vi "GUI.vi"() -> ()   [LabVIEW 2019]
uses:
  Histogram/Histogram.lvlib
panel:
  out "STATUS":u32
  out "BUSY":bool
  in  "CONNECT":bool
  in  "Tab Control":enum32{"ADC and Decimator", "pAmp CTRL"}(tab)
  in  "Full Scale Range":bool
  in  "DDR":bool
  in  "DCLK_RST":bool
  in  "ON":bool=TRUE
  in  "LED 1":bool
  in  "LED 0":bool=TRUE
  in  "CAL":bool
  in  "CAL_DLY":bool
  in  "OUTV":bool
  out "ADC500_CFG":u32=128
  in  "N":u32=100
  out "number":u32=9
  in  "SET POTS":bool
  in  "FINE OFFSET":u16(slide)=1023 scale=0.0..1023.0
  in  "OFFSET":u16(slide)=1023 scale=0.0..1023.0
  in  "HV_CTRL":bool
  out "RANGE 2":bool=TRUE
  out "RANGE 1":bool
  in  "RANGE":bool
  in  "LED":bool=TRUE
  in  "INIT":bool
  out "CONNECTED":bool
  in  "remote port or service name":u16=7
  in  "address":string="10.47.1.10"
  in  "Tab Control 2":T1(tab)
  in  "SET":bool
  in  "TRIGGER_LEVEL":u32=1200
  in  "TRIG_DELAY":u32=500
  in  "FIFO_SIZE":u32=1000
  in  "Trigger Edge":u32(ring)=2 items=["Falling Edge", "Rising Edge", "Auto", "EXT"]
  out "Oscilloscope":u32[](graph)
  in  "CONTINOUS":bool
  in  "Counts":u32
  in  "GEN HISTO":bool
  in  "ENABLE":bool
  out "HISTOGRAM":u32[](graph)
  out "DONE":bool
  out "Progress":u32(slide) max=100000 scale=-1.0..100000.0
  out "IMON GRAPH":dbl(graph)
  out "IMON":fxp<+,16,16>
  out "VMON":fxp<+,32,32>
  in  "VSET":u16
  in  "ON/OFF":bool
  in  "KILL":bool
  in  "TUPRMP":u16
  in  "TDRMP":u16
  out "VMON GRAPH":dbl(graph)
  out "VsetCoeff":dbl
  in  "VMAX":dbl
  out "pAs_STATUS":u8[](array[numeric])=[1, 0, 0, 0, 9, 0, 0, 0]
  out "PAM_INIT_STATUS":u8[](array[numeric])
  out "ADC500_STATUS":u8[](array[numeric])
  out "DEC_STATUS":u8[](array[numeric])
  out "nCoeff":dbl
  out "dacNVSET":u32
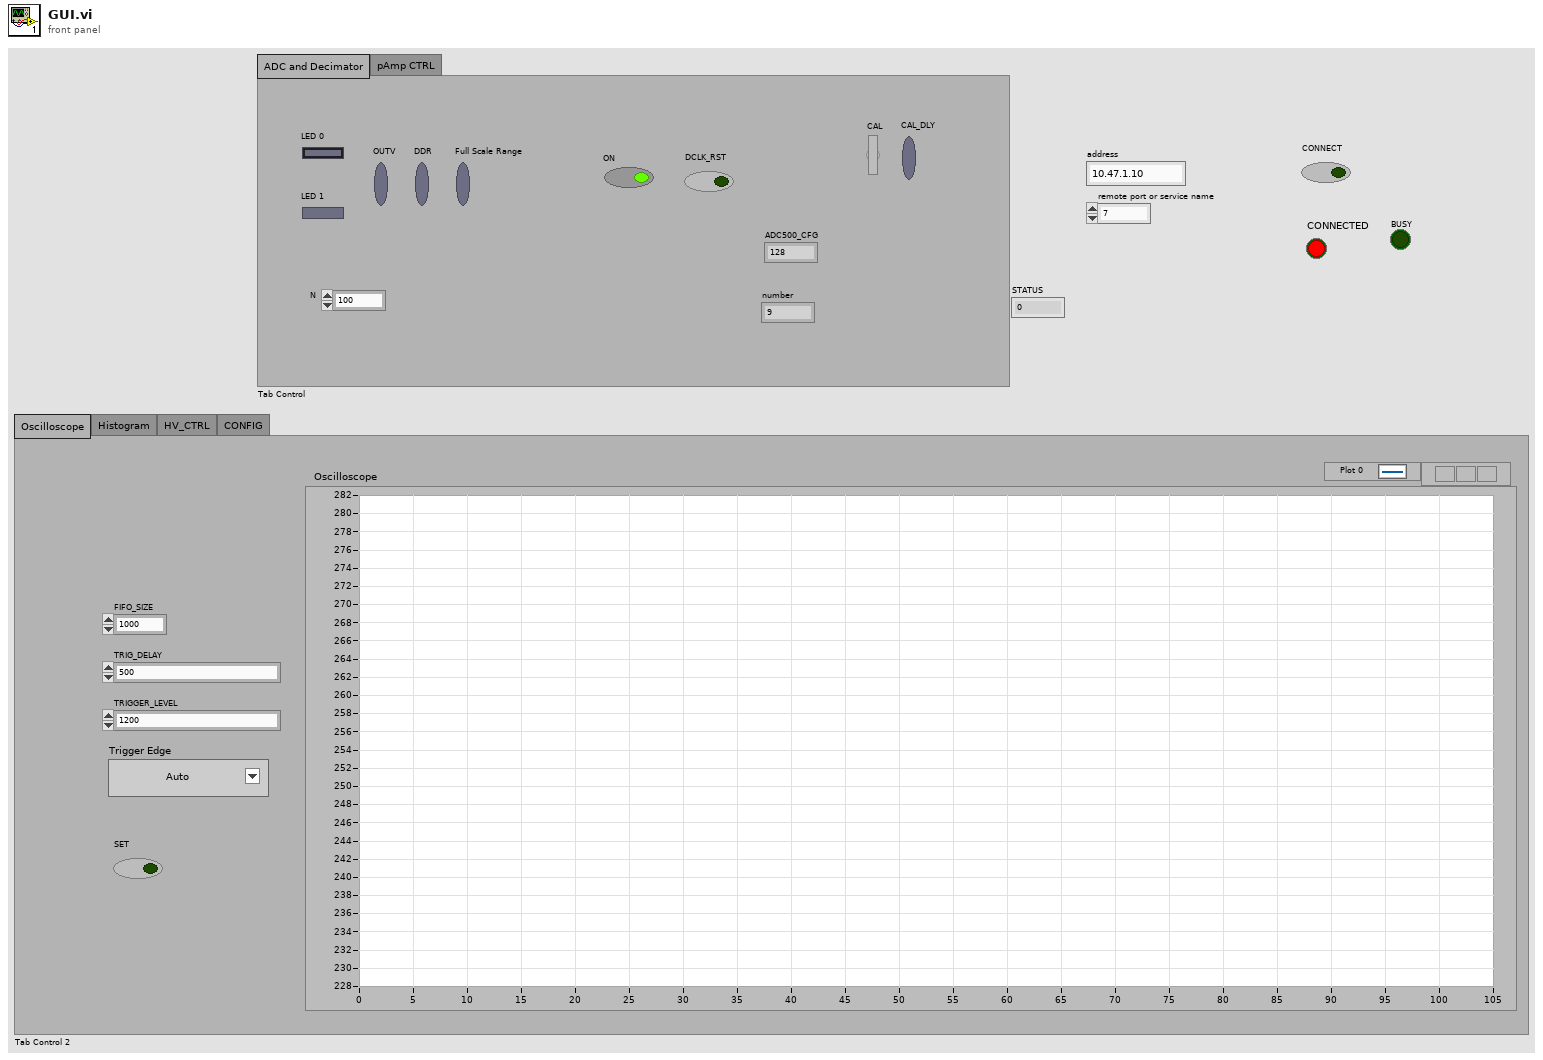
[diagram p1: front panel]
types:
  T1 = enum32{"Oscilloscope", "Histogram", "HV_CTRL", "CONFIG"}
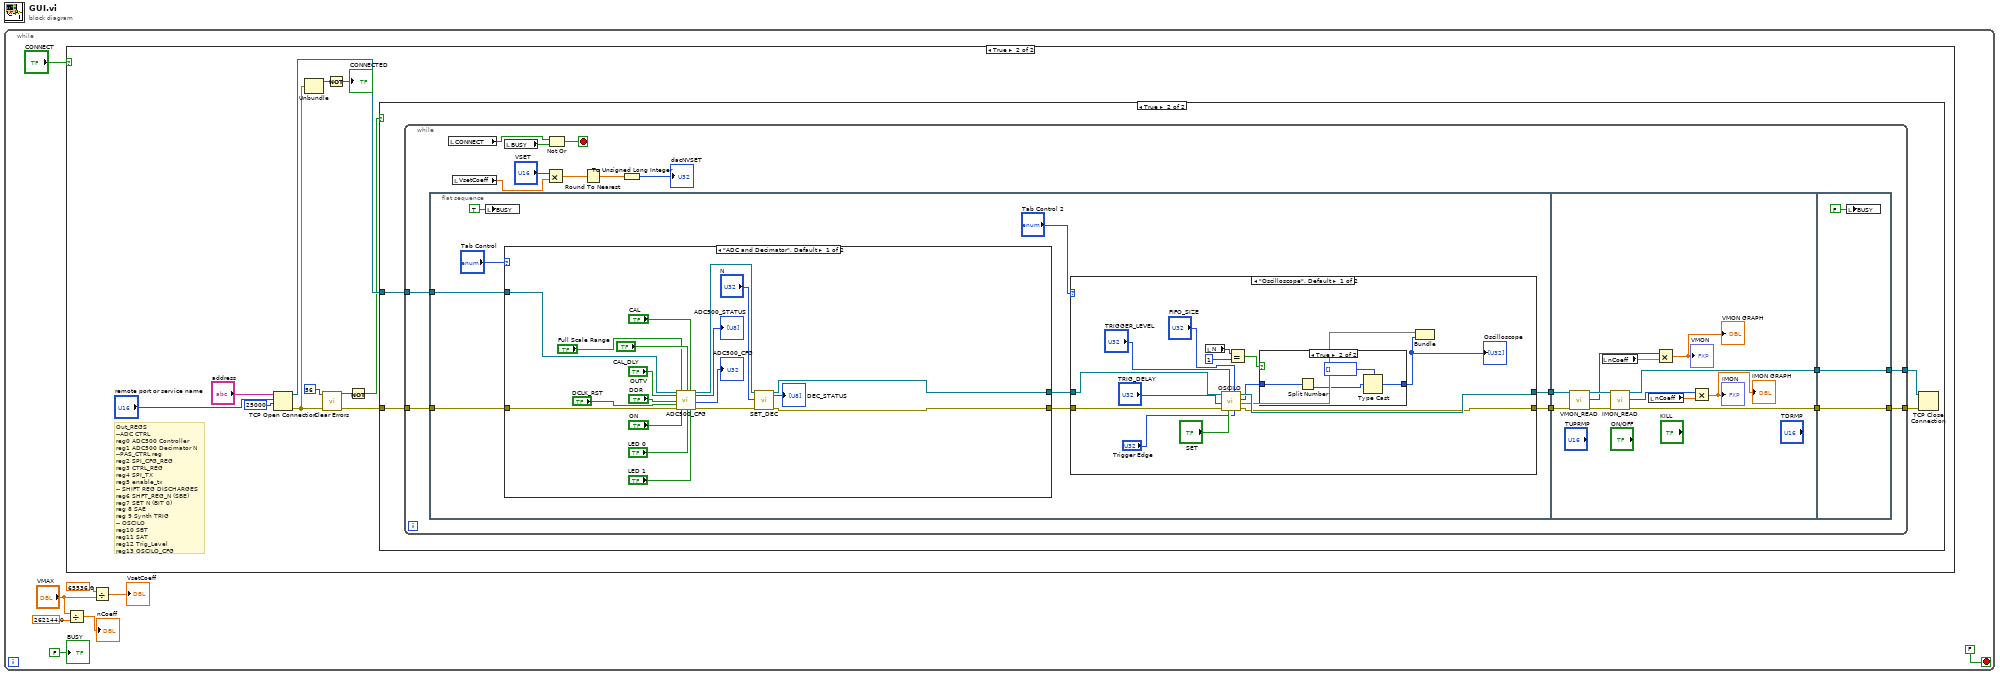
[diagram p0: block diagram]
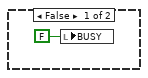
[diagram p3: hidden frame]
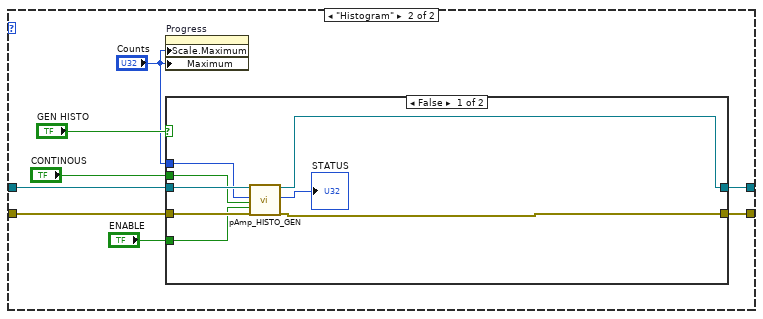
[diagram p5: hidden frame]
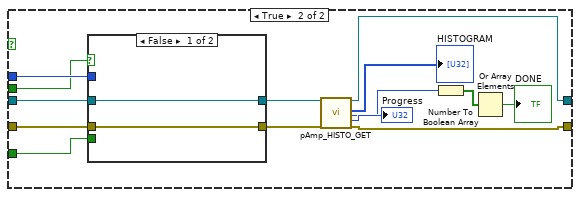
[diagram p6: hidden frame]
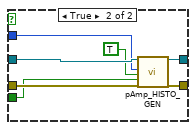
[diagram p7: hidden frame]
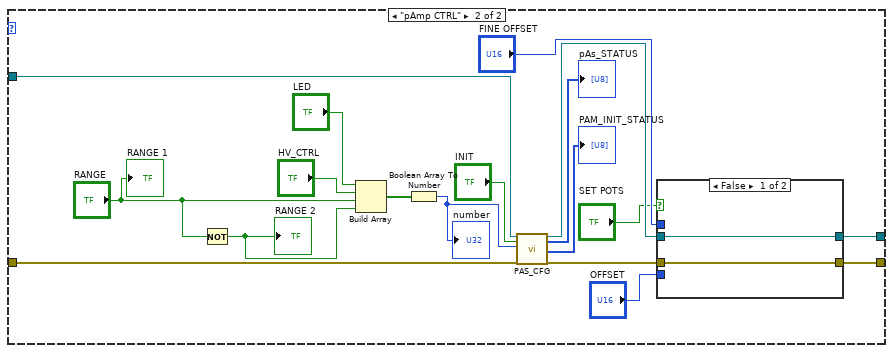
[diagram p8: hidden frame]
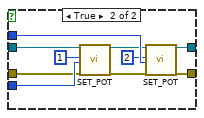
[diagram p9: hidden frame]
diagram:
  n1 = while {
    stop <- FALSE stop-if-true
    n2 = case shown="True" "CONNECT" {
      frame False {
      }
      frame True {
        # "Out_REGS\n--ADC CTRL\nreg0 ADC500 Controller\nreg1 ADC500 Decimator N\n--PAS_CTRL reg\nreg2 SPI_CFG_REG\nreg3 CTRL_REG\nreg4 SPI_TX\nreg5 enable_tx\n-- SHIFT REG DISCHARGES\nreg6 SHFT_REG_N (SBE)\nreg7 SET N (BIT 0)\nreg 8 SAE\nreg 9 Synth TRIG\n-- OSCILO \nreg10 SBT\nreg11 SAT\nreg12 Trig_Level\nreg13 OSCILO_CFG"
        n3 = TCP Open Connection(address="address", remote port or service name="remote port or service name", timeout ms (60000)=25000) -> (connection ID=w19:refnum<k5>, error out=w13:errorcluster)  [unwired: 2 in]
        n4 = Unbundle(w13) -> ("status"=w18:bool)  [unwired: 2 out]
        n5 = call <vilib>:"Clear Errors.vi"("error in (no error)"=w13, "specific error code to clear (0: all)"=56) -> ("error out"=w11:errorcluster, "specific error cleared?"=w10:bool)  [unwired: 4 in]
        n6 = Not(x=w18) -> (.not. x?=→"CONNECTED":bool)
        n7 = Not(x=w10) -> (.not. x?=w9:bool)
        n8 = case shown="True" w9 {
          tunnel: w19 -> [_ w24]
          tunnel: w11 -> [_ w23]
          frame False {
            n9 = local write "BUSY"(FALSE ("BUSY")) -> ()
          }
          frame True {
            n10 = while {
              tunnel: w24 -> [w40]
              tunnel: w23 -> [w39]
              tunnel: [w38] -> w21
              tunnel: [w37] -> w22
              stop <- w34 stop-if-true
              n11 = flat-sequence {
                tunnel: w40 -> [w49]
                tunnel: w39 -> [w48]
                tunnel: [w45] -> w33
                tunnel: [w44] -> w31
                tunnel: w33 -> [w167]
                tunnel: [w169] -> w32
                tunnel: w31 -> [w166]
                tunnel: [w168] -> w30
                tunnel: [w170] -> w37
                tunnel: [w172] -> w38
                tunnel: w32 -> [w172]
                tunnel: w30 -> [w170]
                frame #0 {
                  n12 = local write "BUSY"(TRUE) -> ()
                  n13 = case shown="\"ADC and Decimator\", Default" "Tab Control" {
                    tunnel: [w111 w131] -> w46
                    tunnel: [w109 w129] -> w42
                    tunnel: w48 -> [w127 w139]
                    tunnel: w49 -> [w126 w140]
                    frame "ADC and Decimator", Default {
                      n14 = call "ADC500_CFG.vi"("TCP Network Connection in"=w126, "OUTV"="OUTV", "DDR"="DDR", "DCLK_RST"="DCLK_RST", "error in (no error)"=w127, "Full Scale Range"="Full Scale Range", "ON"="ON", "CAL_DLY"="CAL_DLY", "LED 0"="LED 0", "CAL"="CAL", "LED 1"="LED 1") -> ("TCP Network Connection out"=w114:refnum<k5>, "ADC500_STATUS"=→"ADC500_STATUS":u8[], "ADC500_CFG"=→"ADC500_CFG":u32, "error out"=w112:errorcluster)  [unwired: 5 in]
                      n15 = call "SET_DEC.vi"("TCP Network Connection in"=w114, "N"="N", "error in (no error)"=w112) -> ("TCP Network Connection out"=w111:refnum<k5>, "DEC_STATUS"=→"DEC_STATUS":u8[], "error out"=w109:errorcluster)  [unwired: 14 in]
                    }
                    frame "pAmp CTRL" {
                      n16 = Not(x="RANGE") -> (.not. x?=w142:bool)
                      "RANGE 2" <- w142
                      n17 = Build Array("LED", "HV_CTRL", "RANGE", w142) -> (w141:bool[])
                      n18 = Boolean Array To Number(Boolean array=w141) -> (number=w138:u32)
                      "number" <- w138
                      n19 = call "PAS_CFG.vi"("TCP Network Connection in"=w140, "INIT"="INIT", "pAs_REG"=w138, "error in (no error)"=w139) -> ("TCP Network Connection out"=w132:refnum<k5>, "pAs_STATUS"=→"pAs_STATUS":u8[], "PAM_INIT"=→"PAM_INIT_STATUS":u8[], "error out"=w130:errorcluster)  [unwired: 12 in]
                      n20 = case shown="False" "SET POTS" {
                        tunnel: "OFFSET" -> [_ w157]
                        tunnel: "FINE OFFSET" -> [_ w156]
                        tunnel: w132 -> [w147 w153]
                        tunnel: [w147 w151] -> w131
                        tunnel: w130 -> [w146 w150]
                        tunnel: [w146 w148] -> w129
                        frame False {
                        }
                        frame True {
                          n21 = call "SET_POT.vi"("TCP Network Connection in"=w153, "POT_N"=u32 1, "VALUE"=w157, "error in (no error)"=w150) -> ("TCP Network Connection out"=w152:refnum<k5>, "error out"=w149:errorcluster)  [unwired: 13 in, 1 out]
                          n22 = call "SET_POT.vi"("TCP Network Connection in"=w152, "POT_N"=u32 2, "VALUE"=w156, "error in (no error)"=w149) -> ("TCP Network Connection out"=w151:refnum<k5>, "error out"=w148:errorcluster)  [unwired: 13 in, 1 out]
                        }
                      }
                      "RANGE 1" <- "RANGE"
                    }
                  }
                  n23 = case shown="\"Oscilloscope\", Default" "Tab Control 2" {
                    tunnel: w46 -> [w60 w77]
                    tunnel: [w59 w75] -> w45
                    tunnel: [w58 w74] -> w44
                    tunnel: w42 -> [w57 w76]
                    frame "Oscilloscope", Default {
                      n24 = local read "N"() -> (w54:u32)
                      n25 = call "OSCILO.vi"("Trigger Edge"="Trigger Edge", "FIFO_SIZE"="FIFO_SIZE", "SET"="SET", "TRIGGER_LEVEL"="TRIGGER_LEVEL", "error in (no error)"=w57, "TRIG_DELAY"="TRIG_DELAY", "TCP Network Connection in"=w60) -> ("error out"=w58:errorcluster, 1:w51, "Oscilloscope"=w55:u32[], "TCP Network Connection out"=w59:refnum<k5>)  [unwired: 1 in]
                      n26 = Equal?(x=w54, y=u32 1) -> (x = y?=w52:bool)
                      n27 = case shown="True" w52 {
                        tunnel: [w65 w68] -> w50
                        tunnel: w55 -> [w65 w67]
                        frame False {
                        }
                        frame True {
                          n28 = Split Number(x=w67) -> (lo(x)=w66:u16[])  [unwired: 1 out]
                          n29 = Type Cast(type=i8[] [] ("Oscilloscope"), x=w66) -> (*(type *) &x=w68:i8[])
                        }
                      }
                      "Oscilloscope" <- w50
                      n30 = Bundle(w51, "Oscilloscope"=w50) -> ()  [unwired: 1 in, 1 out]
                    }
                    frame "Histogram" {
                      n31 = property on="Progress" class="Slide (strict)"("Scale.Maximum"="Counts", "Maximum"="Counts") -> ()  [unwired: 2 in, 2 out]
                      n32 = case shown="False" "GEN HISTO" {
                        tunnel: w77 -> [w85 w89]
                        tunnel: w76 -> [w84 w90]
                        tunnel: [w79 w94] -> w75
                        tunnel: [w78 w93] -> w74
                        tunnel: "ENABLE" -> [w80 w86]
                        tunnel: "Counts" -> [w83 w88]
                        tunnel: "CONTINOUS" -> [w82 w87]
                        frame False {
                          n33 = call "pAmp_HISTO_GEN.vi"("TCP Network Connection in"=w85, "COUNTS"=w83, "CONTINOUS"=w82, "ENABLE"=w80, "error in (no error)"=w84) -> ("TCP Network Connection out"=w79:refnum<k5>, "STATUS"=→"STATUS":u32, "error out"=w78:errorcluster)  [unwired: 12 in]
                        }
                        frame True {
                          n34 = case shown="False" w87 {
                            tunnel: [w101 w108] -> w92
                            tunnel: [w100 w107] -> w91
                            tunnel: w90 -> [w100 w105]
                            tunnel: w89 -> [w101 w106]
                            tunnel: w88 -> [_ w104]
                            tunnel: w86 -> [_ w102]
                            frame False {
                            }
                            frame True {
                              n35 = call "pAmp_HISTO_GEN.vi"("TCP Network Connection in"=w106, "COUNTS"=w104, "CONTINOUS"=TRUE, "ENABLE"=w102, "error in (no error)"=w105) -> ("TCP Network Connection out"=w108:refnum<k5>, "error out"=w107:errorcluster)  [unwired: 12 in, 1 out]
                            }
                          }
                          n36 = call "pAmp_HISTO_GET.vi"("TCP Network Connection in"=w92, "error in (no error)"=w91) -> ("TCP Network Connection out"=w94:refnum<k5>, "Oscilloscope"=→"HISTOGRAM":u32[], "DONE"=w97:u32, "CURR_COUNT"=→"Progress":u32, "error out"=w93:errorcluster)  [unwired: 12 in, 1 out]
                          n37 = Number To Boolean Array(number=w97) -> (Boolean array=w96:bool[])
                          n38 = Or Array Elements(Boolean array=w96) -> (logical OR=→"DONE":bool)
                        }
                      }
                    }
                  }
                }
                frame #1 {
                  n39 = call "VMON_READ.vi"("TCP Network Connection in"=w167, "error in (no error)"=w166) -> ("TCP Network Connection out"=w165:refnum<k5>, "VALUE"=w163:u32, "error out"=w164:errorcluster)  [unwired: 14 in, 1 out]
                  n40 = local read "nCoeff"() -> (w162:dbl)
                  n41 = call "IMON_READ.vi"("TCP Network Connection in"=w165, "error in (no error)"=w164) -> ("TCP Network Connection out"=w169:refnum<k5>, "VALUE"=w160:u32, "error out"=w168:errorcluster)  [unwired: 14 in, 1 out]
                  n42 = local read "nCoeff"() -> (w158:dbl)
                  n43 = Multiply(x=w163, y=w162) -> (x*y=→"VMON" →"VMON GRAPH":dbl)
                  n44 = Multiply(x=w160, y=w158) -> (x*y=→"IMON" →"IMON GRAPH":dbl)
                }
                frame #2 {
                  n45 = local write "BUSY"(FALSE) -> ()
                }
              }
              n46 = local read "CONNECT"() -> (w36:bool)
              n47 = local read "VsetCoeff"() -> (w26:dbl)
              n48 = local read "BUSY"() -> (w35:bool)
              n49 = Multiply(x="VSET", y=w26) -> (x*y=w28:dbl)
              n50 = Not Or(1:w35, 2:w36) -> (0:w34:bool)
              n51 = Round To Nearest(number=w28) -> (nearest integer value=w27:dbl)
              n52 = To Unsigned Long Integer(number=w27) -> (unsigned 32bit integer=→"dacNVSET":u32)
            }
            n53 = TCP Close Connection(connection ID=w21, error in (no error)=w22) -> ()  [unwired: 1 in, 2 out]
          }
        }
      }
    }
    n54 = Divide(x="VMAX", y=262144.0) -> (x/y=→"nCoeff":dbl)
    n55 = Divide(x=65536.0 ("y"), y="VMAX") -> (x/y=→"VsetCoeff":dbl)
    "BUSY" <- FALSE ("BUSY")
  }
